vi "Event Log.vi"(8 "Event Type":string, 9 "Message":string, 10 "Location":string) -> ()   [LabVIEW 2024, in "Sift TDMS Uploader.lvlib" / "Sift TDMS Uploader.lvclass"]
uses:
  Sift TDMS Uploader.lvclass
panel:
  in  "error in (no error)":errorcluster
  out "error out":errorcluster
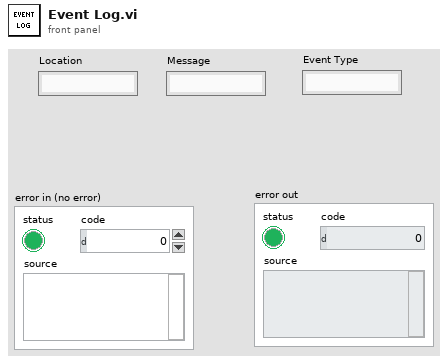
[diagram p1: front panel]
types:
  T1 = enum16{"open", "replace", "create", "open or create", "replace or create", "replace or create with confirmation"}
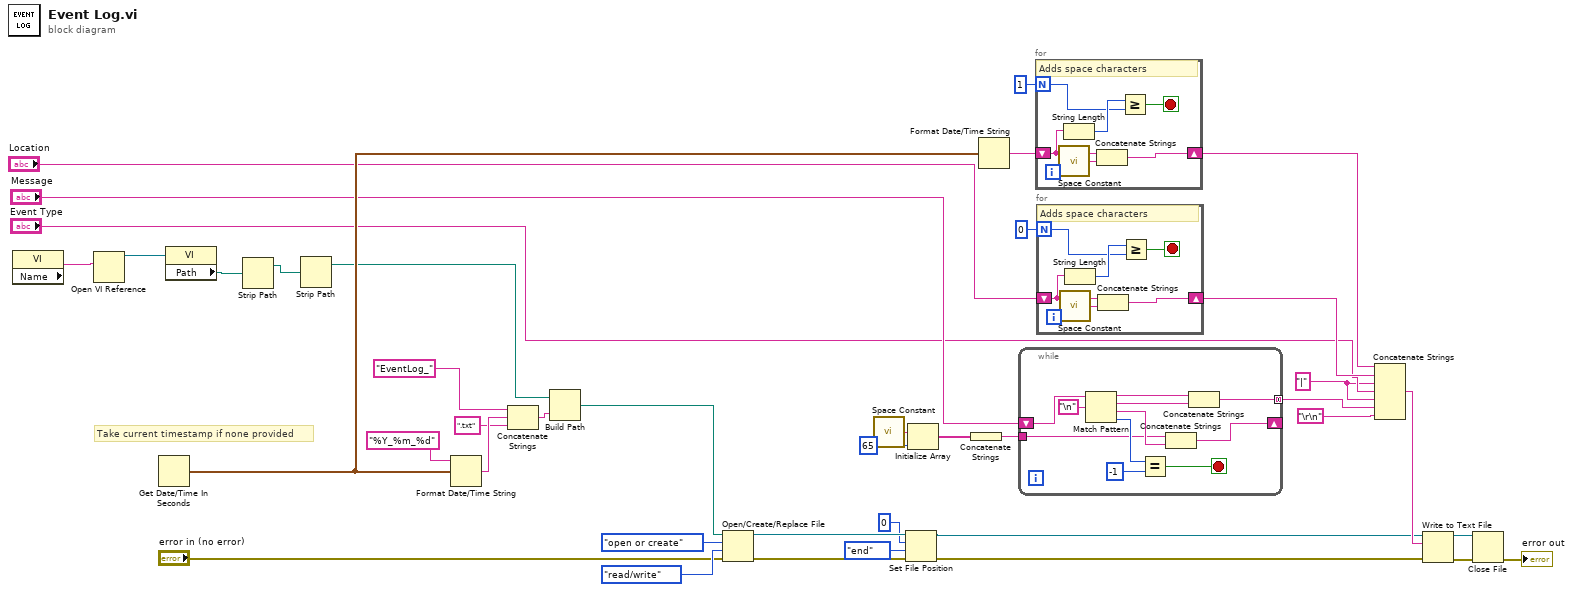
[diagram p0: block diagram]
diagram:
  w3 = "|" ("string")
  # "Take current timestamp if none provided"
  n1 = property class="VI"() -> ("Name"=w9:string)  [unwired: 2 in, 2 out]
  n2 = Open VI Reference(vi path=w9) -> (vi reference=w11:refnum<vi>)  [unwired: 5 in, 1 out]
  n3 = Get Date/Time In Seconds() -> (seconds since 1Jan1904=w13:timestamp)
  n4 = property class="VI"(reference=w11) -> ("Path"=w10:path)  [unwired: 1 in, 2 out]
  n5 = Strip Path(path=w10) -> (stripped path=w2:path)  [unwired: 1 out]
  n6 = Strip Path(path=w2) -> (stripped path=w1:path)  [unwired: 1 out]
  n7 = Format Date/Time String(time format string (%c)="%Y_%m_%d", seconds (now)=w13) -> (date/time string=w28:string)  [unwired: 1 in]
  n8 = Concatenate Strings("EventLog_" ("string"), w28, ".txt" ("string")) -> (w27:string)
  n9 = Build Path(base path=w1, name or relative path=w27) -> (appended path=w14:path)
  n10 = Open/Create/Replace File(file path (use dialog)=w14, error in="error in (no error)", operation (0:open)=T1."open or create", access (0:read/write)=enum16{"read/write", "read-only", "write-only"}."read/write") -> (refnum out=w23:refnum<file>, error out=w24:errorcluster)  [unwired: 2 in, 1 out]
  n11 = call <vilib>:"Space Constant.vi"() -> ("String"=w34:string)
  n12 = Set File Position(offset (in bytes) (0)=i64 0, refnum=w23, from (0:start)=enum16{"start", "end", "current"}."end", error in=w24) -> (refnum out=w15:refnum<file>, error out=w19:errorcluster)
  n13 = Initialize Array(w34, 65 ("dimension size")) -> (w32:string[])
  n14 = Concatenate Strings(w32) -> (w31:string)
  n15 = Format Date/Time String(seconds (now)=w13) -> (date/time string=w37:string)  [unwired: 2 in]
  n16 = while {
    shift-right: [w44] -> _
    shift-left: "Message" -> [w47]
    tunnel: w31 -> [w45]
    tunnel: [w41] -> w5 mode=concatenating
    stop <- w48 stop-if-true
    n17 = Match Pattern(string=w47, regular expression="\n") -> (before substring=w43:string, match substring=w42:string, after substring=w46:string, offset past match=w49:i32)  [unwired: 1 in]
    n18 = Equal?(x=w49, y=-1) -> (x = y?=w48:bool)
    n19 = Concatenate Strings(w45, w46) -> (w44:string)
    n20 = Concatenate Strings(w43, w42) -> (w41:string)
  }
  n21 = for {
    N: 1 -> [w52]
    shift-right: [w54] -> w36
    shift-left: w37 -> [w57]
    stop <- w53 stop-if-true
    # "Adds space characters"
    n22 = call <vilib>:"Space Constant.vi"() -> ("String"=w55:string)
    n23 = String Length(string=w57) -> (length=w56:i32)
    n24 = Concatenate Strings(w57, w55) -> (w54:string)
    n25 = Greater Or Equal?(x=w56, y=w52) -> (x >= y?=w53:bool)
  }
  n26 = for {
    N: 0 -> [w58]
    shift-right: [w60] -> w35
    shift-left: "Location" -> [w63]
    stop <- w59 stop-if-true
    # "Adds space characters"
    n27 = call <vilib>:"Space Constant.vi"() -> ("String"=w61:string)
    n28 = String Length(string=w63) -> (length=w62:i32)
    n29 = Concatenate Strings(w63, w61) -> (w60:string)
    n30 = Greater Or Equal?(x=w62, y=w58) -> (x >= y?=w59:bool)
  }
  n31 = Concatenate Strings(w36, w35, w3, "Event Type", w3, w5, "\r\n") -> (w40:string)
  n32 = Write to Text File(file (use dialog)=w15, text=w40, error in=w19) -> (refnum out=w18:refnum<file>, error out=w17:errorcluster)  [unwired: 1 in, 1 out]
  n33 = Close File(refnum=w18, error in=w17) -> (error out=→"error out":errorcluster)  [unwired: 1 out]
